vi "Init.vi"(8 "error in (no error)":errorcluster, 10 "Channel":i16, 11 "TrialBasedExperiment in":refnum<class "CenterSurround.lvclass">) -> (0 "error out":errorcluster, 3 "TrialBasedExperiment out":refnum<class "CenterSurround.lvclass">)   [LabVIEW 2014, in "CenterSurround.lvclass"]
uses:
  CenterSurround.lvclass
  Trial Based Experiment Statechart/PassiveExperiment/PassiveExperiment.lvclass
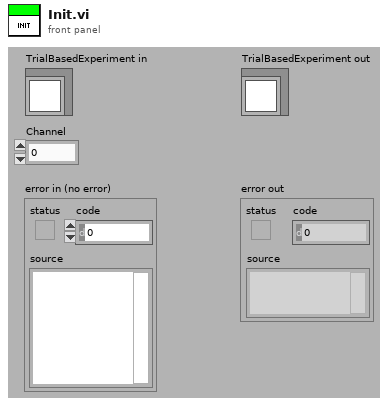
[diagram p1: front panel]
types:
  T1 = cluster{"Intertrial":dbl, "AcquireFixation":dbl, "HoldFixation":dbl, "DelayPeriod":dbl, "ResponsePeriod":dbl}
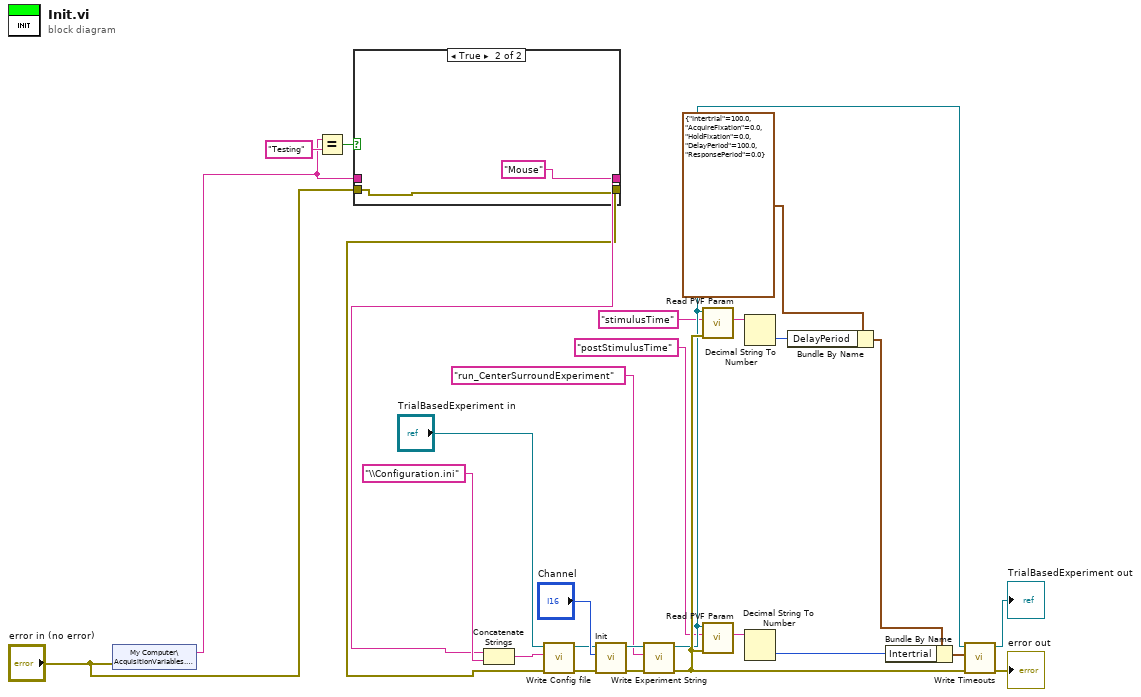
[diagram p0: block diagram]
diagram:
  n1 = shared-variable "My Computer\\AcquisitionVariables.lvlib\\Subject"(error in="error in (no error)") -> (w4:string)  [unwired: 1 out]
  n2 = Equal?(x=w4, y="Testing") -> (x = y?=w5:bool)
  n3 = case shown="True" w5 {
    tunnel: [w30 "Mouse" ("String")] -> w2
    tunnel: w4 -> [w30 _]
    tunnel: "error in (no error)" -> [w29 w32]
    tunnel: [w29 w32] -> w1
    frame False {
    }
    frame True {
    }
  }
  n4 = Concatenate Strings(w2, "\\Configuration.ini") -> (w11:string)
  n5 = call-dynamic "Write Config file.vi"("error in (no error)"=w1, "Config file"=w11, "TrialBasedExperiment in"="TrialBasedExperiment in") -> ("error out"=w7:errorcluster, "TrialBasedExperiment out"=w8:refnum<class "CenterSurround.lvclass">)  [unwired: 7 in]
  n6 = call-parent "Init.vi"("error in (no error)"=w7, "Channel"="Channel", "TrialBasedExperiment in"=w8) -> ("error out"=w15:errorcluster, "TrialBasedExperiment out"=w16:refnum<class "CenterSurround.lvclass">)  [unwired: 7 in]
  n7 = call-dynamic "Write Experiment String.vi"("error in (no error)"=w15, "Experiment String"="run_CenterSurroundExperiment" ("string"), "TrialBasedExperiment in"=w16) -> ("error out"=w25:errorcluster, "TrialBasedExperiment out"=w24:refnum<class "CenterSurround.lvclass">)  [unwired: 7 in]
  n8 = call-dynamic "Read PVF Param.vi"("error in (no error)"=w25, "Param Name"="stimulusTime", "MatlabExperiment in"=w24) -> ("Param Value"=w19:string)  [unwired: 6 in, 2 out]
  n9 = call-dynamic "Read PVF Param.vi"("error in (no error)"=w25, "Param Name"="postStimulusTime", "MatlabExperiment in"=w24) -> ("Param Value"=w22:string)  [unwired: 6 in, 2 out]
  n10 = Decimal String To Number(string=w19) -> (number=w20:i32)  [unwired: 2 in, 1 out]
  n11 = Decimal String To Number(string=w22) -> (number=w23:i32)  [unwired: 2 in, 1 out]
  n12 = Bundle By Name(cluster=T1 {"Intertrial"=100.0, "AcquireFixation"=0.0, "HoldFixation"=0.0, "DelayPeriod"=100.0, "ResponsePeriod"=0.0} ("Timeouts"), "DelayPeriod"=w20) -> (w26:T1)
  n13 = Bundle By Name(cluster=w26, "Intertrial"=w23) -> (w27:T1)
  n14 = call-dynamic "Write Timeouts.vi"("error in (no error)"=w25, "Timeouts"=w27, "TrialBasedExperiment in"=w24) -> ("error out"=→"error out":errorcluster, "TrialBasedExperiment out"=→"TrialBasedExperiment out":refnum<class "CenterSurround.lvclass">)  [unwired: 7 in]
